vi "Fly.vi"(8 "error in (no error)":errorcluster caption="错误输入（无错误）", 10 "字符串":string, 11 "Hummingbird 输入":refnum<class "Hummingbird.lvclass">) -> (0 "error out":errorcluster caption="错误输出", 2 "字符串 2":string, 3 "Hummingbird 输出":refnum<class "Hummingbird.lvclass">)   [LabVIEW 2020, in "Hummingbird.lvclass"]
uses:
  Hummingbird.lvclass
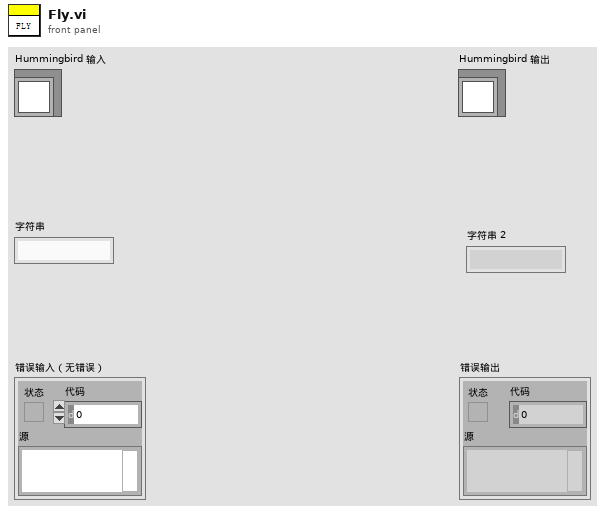
[diagram p1: front panel]
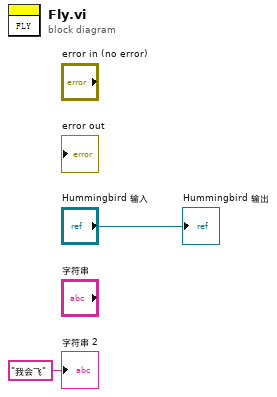
[diagram p0: block diagram]
diagram:
  "Hummingbird 输出" <- "Hummingbird 输入"
  "字符串 2" <- "我会飞" ("字符串 2")
